vi "Peak_Comparator.vi"(7 "threshold":dbl, 10 "Detected peaks":T1[][](array[typedef]), 11 "Reference peaks":T1[][](array[typedef])) -> (2 "Przekroczenia":string[][](array[string]), 3 "Alarm?":bool[](array[boolean]))   [LabVIEW 2021]
uses:
  Typedefs/Detected peaks.ctl
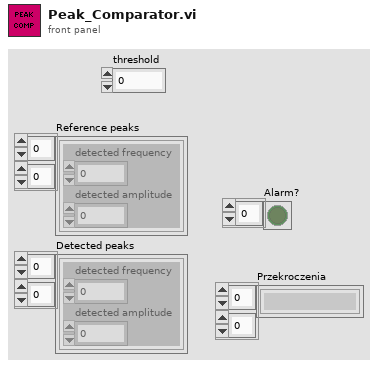
[diagram p1: front panel]
types:
  T1 = typedef "Detected peaks.ctl" = cluster{"detected frequency":dbl, "detected amplitude":dbl}
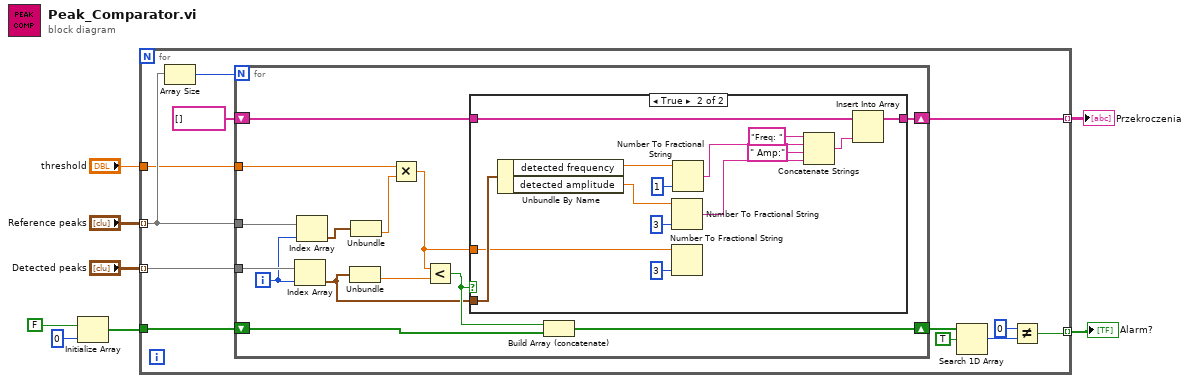
[diagram p0: block diagram]
diagram:
  n1 = Initialize Array(FALSE, 0 ("dimension size")) -> (w6:bool[])
  n2 = for {
    tunnel: "Reference peaks" -> [w17] mode=indexing
    tunnel: "Detected peaks" -> [w20] mode=indexing
    tunnel: w6 -> [w19]
    tunnel: [w11] -> w2 mode=indexing
    tunnel: "threshold" -> [w16]
    tunnel: [w9] -> w1 mode=indexing
    n3 = Array Size(array=w17) -> (size(s)=w18:i32)
    n4 = for {
      N: w18 -> [_]
      tunnel: w17 -> [w33]
      tunnel: w20 -> [w34]
      shift-right: [w28] -> w15
      shift-left: w19 -> [w29]
      tunnel: w16 -> [w27]
      shift-right: [w22] -> w9
      shift-left: string[] [] -> [w21]
      i -> [w32]
      n5 = Index Array(array=w34, index=w32) -> (element=w25:T1)
      n6 = Index Array(array=w33, index=w32) -> (element=w24:T1)
      n7 = Unbundle(w25) -> ("detected amplitude"=w30:dbl)  [unwired: 1 out]
      n8 = Unbundle(w24) -> ("detected amplitude"=w31:dbl)  [unwired: 1 out]
      n9 = Multiply(x=w27, y=w31) -> (x*y=w23:dbl)
      n10 = Less?(x=w23, y=w30) -> (x < y?=w26:bool)
      n11 = case shown="True" w26 {
        tunnel: w25 -> [_ w49]
        tunnel: w23 -> [_ w42]
        tunnel: [w35 w40] -> w22
        tunnel: w21 -> [w35 w39]
        frame False {
        }
        frame True {
          n12 = Unbundle By Name(w49) -> ("detected frequency"=w48:dbl, "detected amplitude"=w47:dbl)
          n13 = Number To Fractional String(number=w47, precision (6)=i16 3) -> (F-format string=w43:string)  [unwired: 2 in]
          n14 = Number To Fractional String(number=w42, precision (6)=i16 3) -> ()  [unwired: 2 in, 1 out]
          n15 = Number To Fractional String(number=w48, precision (6)=i16 1) -> (F-format string=w46:string)  [unwired: 2 in]
          n16 = Concatenate Strings("Freq: " ("string"), w46, " Amp:" ("string"), w43) -> (w41:string)
          n17 = Insert Into Array(array=w39, new element=w41) -> (w40:string[])  [unwired: 1 in]
        }
      }
      n18 = Build Array (concatenate)(w26, w29) -> (w28:bool[])
    }
    n19 = Search 1D Array(1D array=w15, element=TRUE) -> (index of element=w13:i32)  [unwired: 1 in]
    n20 = Not Equal?(x=0, y=w13) -> (x != y?=w11:bool)
  }
  "Alarm?" <- w2
  "Przekroczenia" <- w1
